vi "Set Line Style.vi"(6 "Weight (pt)":sgl, 8 "error in (no error)":errorcluster, 9 "Color":u32(colorbox), 10 "Shape refnum":refnum<k7>) -> (0 "error out":errorcluster, 2 "reference out":refnum<k7>)   [LabVIEW 2020, in "lvpptx.lvlib"]
uses:
  lvpptx.lvlib
panel:
  # "If weight <= 0, borders will be invisible"
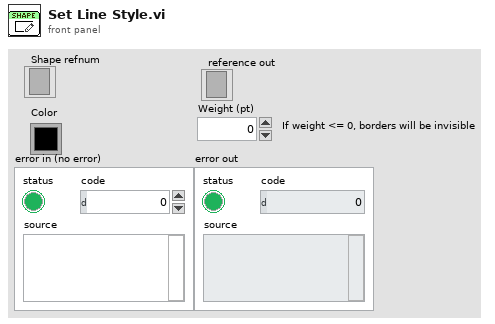
[diagram p1: front panel]
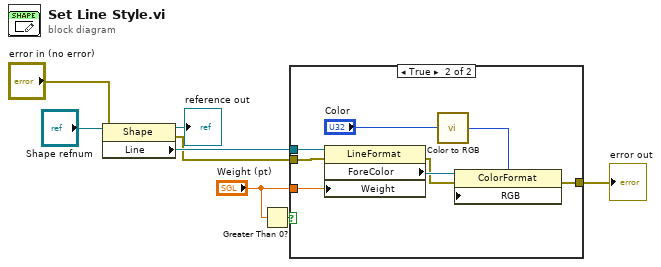
[diagram p0: block diagram]
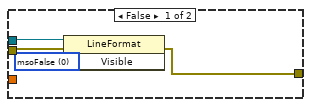
[diagram p2: hidden frame]
diagram:
  n1 = property class="Shape"(reference="Shape refnum", error in="error in (no error)") -> (reference out=→"reference out":refnum<k7>, error out=w1:errorcluster, "Line"=w4:refnum<k7>)
  n2 = Greater Than 0?(x="Weight (pt)") -> (x > 0?=w3:bool)
  n3 = case shown="True" w3 {
    tunnel: [w10 w16] -> w5
    tunnel: w4 -> [w12 w15]
    tunnel: "Weight (pt)" -> [_ w14]
    tunnel: w1 -> [w11 w13]
    frame False {
      w9 = 0 items=["msoTrue"=-1, "msoFalse"=0, "msoCTrue"=1, "msoTriStateToggle"=-3, "msoTriStateMixed"=-2] ("Visible")
      n4 = property class="LineFormat"(reference=w12, error in=w11, "Visible"=w9) -> (error out=w10:errorcluster)  [unwired: 1 out]
    }
    frame True {
      n5 = property class="LineFormat"(reference=w15, error in=w13, "Weight"=w14) -> (error out=w17:errorcluster, "ForeColor"=w20:refnum<k7>)  [unwired: 1 out]
      n6 = call "Color to RGB.vi"("Color"="Color") -> ("32bit out"=w19:u32)  [unwired: 4 in]
      n7 = property class="ColorFormat"(reference=w20, error in=w17, "RGB"=w19) -> (error out=w16:errorcluster)  [unwired: 1 out]
    }
  }
  "error out" <- w5
